vi "Find Multiple Items.vi"(7 "$Path or Item Name":string, 8 "error in (no error)":errorcluster, 10 "Offset":i32, 11 "JSON":string) -> (0 "error out":errorcluster, 1 "<JSON>":string[](array[string]) caption="<JSON>Items", 2 "Item Offsets":i32[](array[numeric]), 3 "Item Names":string[](array[string]))   [LabVIEW 2021, in "jsontext.facade.lvlib"]
doc: "Find the JSON items at the JSON Path specified and returns them as an array.\n\nPaths specify an item in a tree of nested Elements, and start with $. Each element is either in the form .name, for Object items, or [n] for Array index ([*] for all elements). Multiple Object items can be specified by the list form .[abc,def].\n\nIf the Path input does not start with a $, then it is interpreted as a single Object Item name, rather than a path.\n\nExample JSON:\n{\"A\":[{\"C\":123,\"D\":4},{\"C\":567,\"D\":8}],\"B\":{\"F\":9},\"E\":true}\nAt path $.A[*].C are 123 and 567\nAt path $.B (or just B) is {\"F\":9}\nAt path $.B.F is 9\nAt path $.[B,E] are {\"F\":9} and true"
uses:
  jsontext.facade.lvlib
  jsontext/String Subset.vi
  jsontext/support/Strip Quotes and Unescape.vi
  jsontext/support/Unescape JSON string.vi
  jsontext/Parsing/Parse Full Path or Item Name.vi
  jsontext/Offset/Find Item Locations by Path.vi
  jsontext/JSONtext.lvlib
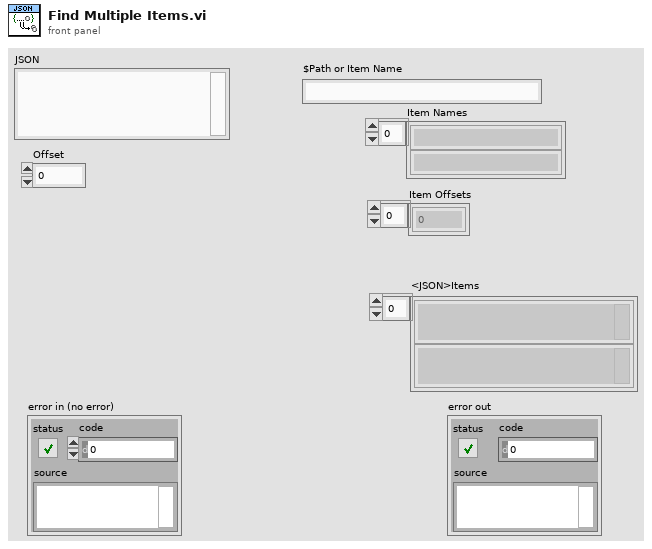
[diagram p1: front panel]
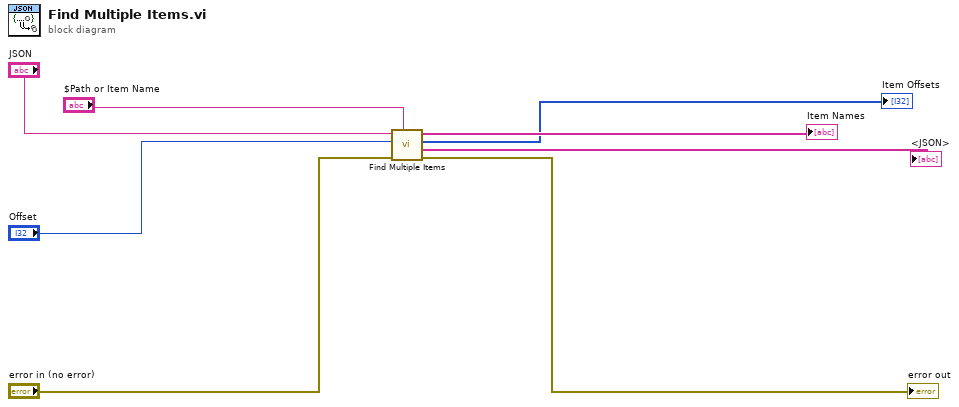
[diagram p0: block diagram]
diagram:
  n1 = call "Find Multiple Items.vi"("$Path or Item Name"="$Path or Item Name", "error in (no error)"="error in (no error)", "Offset"="Offset", "JSON"="JSON") -> ("error out"=→"error out":errorcluster, "<JSON>"=→"<JSON>":string[], "Item Offsets"=→"Item Offsets":i32[], "Item Names"=→"Item Names":string[])  [unwired: 4 in]
